vi "setTargetState (byObject).vi"(8 "error in (no error)":errorcluster, 10 "Target State":refnum<class "state.lvclass">, 11 "statemachine":refnum<class "statemachine.lvclass">) -> (0 "error out":errorcluster, 3 "statemachine out":refnum<class "statemachine.lvclass">)   [LabVIEW 2020, in "eos.lvlib" / "statemachine.lvclass"]
uses:
  statemachine.lvclass
  interfaces/state/state.lvclass
  statemachine.lvclass/statemachine.ctl
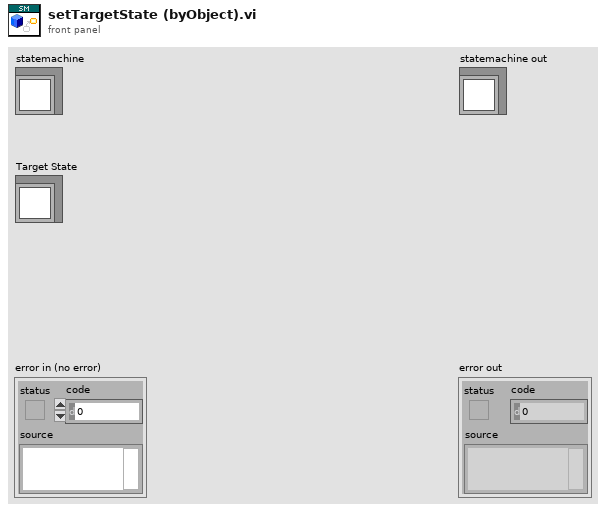
[diagram p1: front panel]
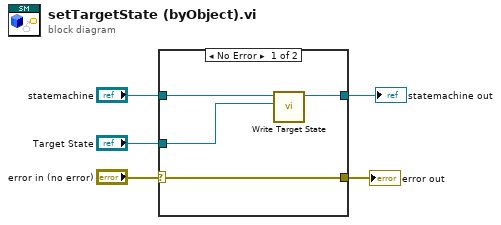
[diagram p0: block diagram]
diagram:
  n1 = case shown="No Error" "error in (no error)" {
    selector: "error in (no error)" -> [w6 w10]
    tunnel: "Target State" -> [w9 _]
    tunnel: "statemachine" -> [w8 w11]
    tunnel: [w7 w11] -> w3
    tunnel: [w6 w10] -> w1
    frame No Error {
      n2 = call "Write Target State.vi"("Target State"=w9, "statemachine in"=w8) -> ("statemachine out"=w7:refnum<class "statemachine.lvclass">)  [unwired: 9 in]
    }
    frame Error {
    }
  }
  "error out" <- w1
  "statemachine out" <- w3
